vi "dvp Vi Get Roi State.vi"(10 "pRoiState":i32, 11 "handle":u32) -> (2 "pRoiState out":i32, 3 "function return":u32(ring))   [LabVIEW 2018, in "LabViewDVPCamera.lvlib"]
doc: "LabviewDvp2Api dvpStatus dvpViGetRoiState(dvpHandle handle, BOOL *pRoiState);"
uses:
  LabViewDVPCamera.lvlib
  LabViewDVPCamera/LabViewDVPCamera.dll
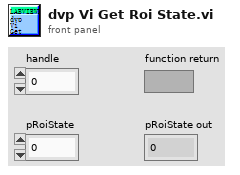
[diagram p1: front panel]
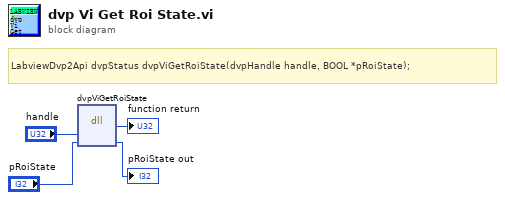
[diagram p0: block diagram]
diagram:
  # "LabviewDvp2Api dvpStatus dvpViGetRoiState(dvpHandle handle, BOOL *pRoiState);"
  n1 = dll-call lib="C:/Program Files (x86)/DVP2 Labview cn 64/Sample/LabViewDVPCamera/LabViewDVPCamera.*" fn="dvpViGetRoiState"("handle"="handle", "pRoiState"="pRoiState") -> (→"function return":u32, "pRoiState"=→"pRoiState out":i32)  [unwired: 4 in, 2 out]
